vi "StringToNumberControlWithBool(x2).vi"(7 "Seperator":string=";", 9 "string":string) -> (0 "Num(2)":dbl, 1 "Num":dbl, 2 "NOT_0(2)":bool, 3 "NOT_0?":bool, 4 "after substring":string, 5 "before substring":string, 6 "Seperator Out":string=";")   [LabVIEW 2018]
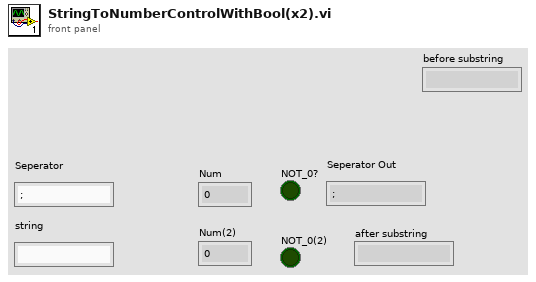
[diagram p1: front panel]
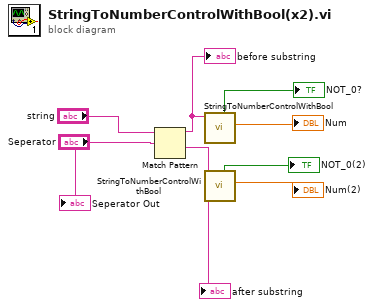
[diagram p0: block diagram]
diagram:
  n1 = Match Pattern(string="string", regular expression="Seperator") -> (before substring=w6:string, after substring=w8:string)  [unwired: 1 in, 2 out]
  "after substring" <- w8
  "before substring" <- w6
  n2 = call "StringToNumberControlWithBool.vi"("String In"=w6) -> ("Number Out"=→"Num":dbl, "NOT = 0"=→"NOT_0?":bool)  [unwired: 7 in]
  n3 = call "StringToNumberControlWithBool.vi"("String In"=w8) -> ("Number Out"=→"Num(2)":dbl, "NOT = 0"=→"NOT_0(2)":bool)  [unwired: 7 in]
  "Seperator Out" <- "Seperator"
